vi "Adquirir Parametro Meteorologico.vi"(8 "error in":errorcluster, 11 "queue in":refnum<queue>) -> (0 "error out":errorcluster, 3 "queue out":refnum<queue>)   [LabVIEW 2015]
uses:
  ClusterM1.ctl
panel:
  out "TEMP SUP.":dbl
  out "HUMED":dbl
  out "RAD":dbl
  out "TEMP AMBIENTE":dbl
  out "AI3":dbl
  out "AI2":dbl
  out "AI1":dbl
  out "AI0":dbl
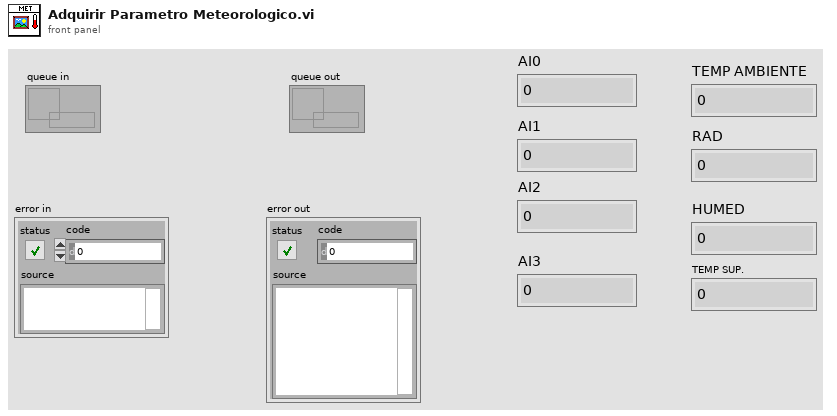
[diagram p1: front panel]
types:
  T1 = typedef "ClusterM1.ctl" = cluster{"group":string, "timeStamp":timestamp, "Temperature Ambient":dbl, "radiation":dbl, "RH":dbl, "Temperature Panel":dbl}
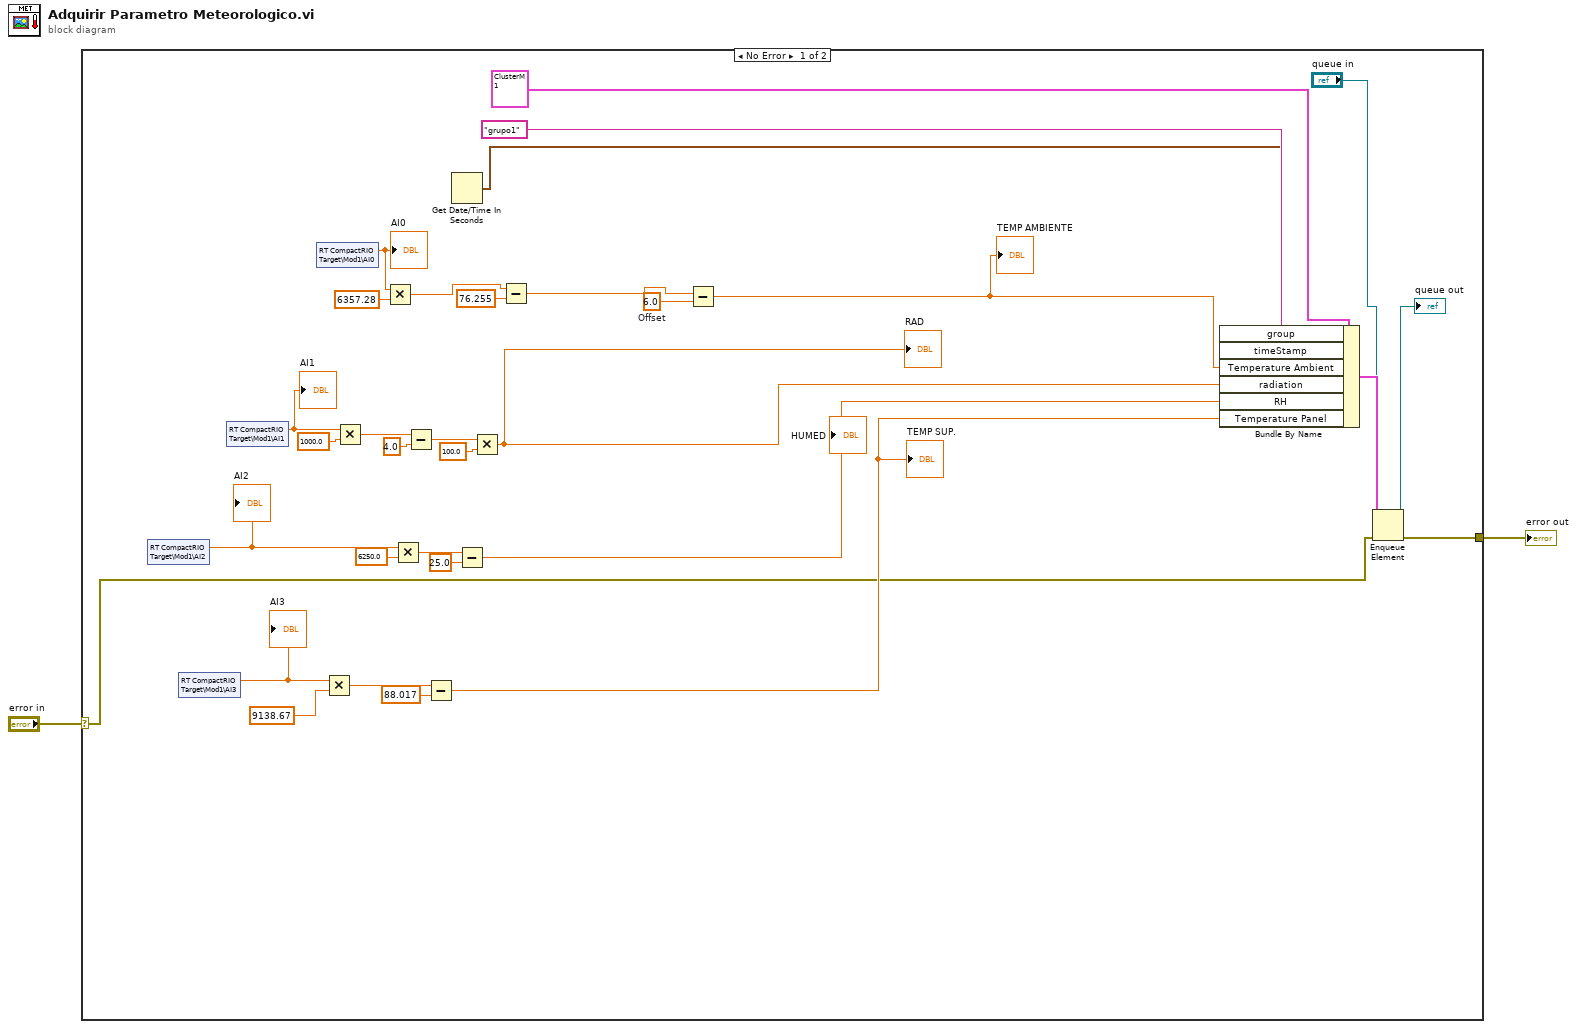
[diagram p0: block diagram]
diagram:
  n1 = case shown="No Error" "error in" {
    selector: "error in" -> [w7 w35]
    tunnel: [w8 w35] -> w1
    frame No Error {
      w5 = 6.0  # Offset
      n2 = shared-variable "RT CompactRIO Target\\Mod1\\AI2"() -> (w21:dbl)  [unwired: 1 in, 1 out]
      "AI2" <- w21
      n3 = shared-variable "RT CompactRIO Target\\Mod1\\AI3"() -> (w16:dbl)  [unwired: 1 in, 1 out]
      "AI3" <- w16
      n4 = shared-variable "RT CompactRIO Target\\Mod1\\AI1"() -> (w31:dbl)  [unwired: 1 in, 1 out]
      "AI1" <- w31
      n5 = shared-variable "RT CompactRIO Target\\Mod1\\AI0"() -> (w6:dbl)  [unwired: 1 in, 1 out]
      "AI0" <- w6
      n6 = Multiply(x=w16, y=9138.67) -> (x*y=w14:dbl)
      n7 = Multiply(x=w31, y=1000.0) -> (x*y=w29:dbl)
      n8 = Multiply(x=w6, y=6357.28) -> (x*y=w23:dbl)
      n9 = Multiply(x=w21, y=6250.0) -> (x*y=w19:dbl)
      n10 = Subtract(x=w29, y=4.0) -> (x-y=w27:dbl)
      n11 = Subtract(x=w14, y=88.017) -> (x-y=w12:dbl)
      "TEMP SUP." <- w12
      n12 = Get Date/Time In Seconds() -> (seconds since 1Jan1904=w32:timestamp)
      n13 = Subtract(x=w19, y=25.0) -> (x-y=w17:dbl)
      "HUMED" <- w17
      n14 = Multiply(x=w27, y=100.0) -> (x*y=w25:dbl)
      "RAD" <- w25
      n15 = Subtract(x=w23, y=76.255) -> (x-y=w4:dbl)
      n16 = Subtract(x=w4, y=w5) -> (x-y=w3:dbl)
      "TEMP AMBIENTE" <- w3
      n17 = Bundle By Name(cluster=T1 {"group"="", "timeStamp"=timestamp(0 s since 1904-01-01), "Temperature Ambient"=0.0, "radiation"=0.0, "RH"=0.0, "Temperature Panel"=0.0} ("M1"), "group"="grupo1", "timeStamp"=w32, "Temperature Ambient"=w3, "radiation"=w25, "RH"=w17, "Temperature Panel"=w12) -> (w11:T1)
      n18 = Enqueue Element(queue="queue in", element=w11, error in (no error)=w7) -> (queue out=→"queue out":refnum<queue>, error out=w8:errorcluster)  [unwired: 1 in, 1 out]
    }
    frame Error {
    }
  }
  "error out" <- w1
